vi "BRig_dataMTrig_Audio_N_R.vi"() -> (2 "output_Audio_N_R":i32)   [LabVIEW 2014]
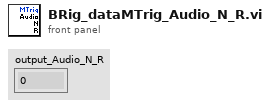
[diagram p1: front panel]
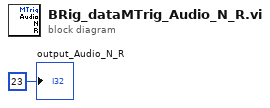
[diagram p0: block diagram]
diagram:
  "output_Audio_N_R" <- 23 ("output_iBlock")
